vi "sub_create_buf_file_from_date.vi"(8 "error in (no error)":errorcluster) -> (0 "error out":errorcluster, 2 "new file path":path, 3 "File Refnum":refnum<file>)   [LabVIEW 2013, in "daqio minimal.lvlib"]
uses:
  daqio minimal.lvlib
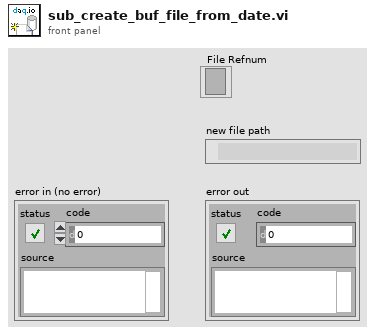
[diagram p1: front panel]
types:
  T1 = enum16{"open", "replace", "create", "open or create", "replace or create", "replace or create with confirmation"}
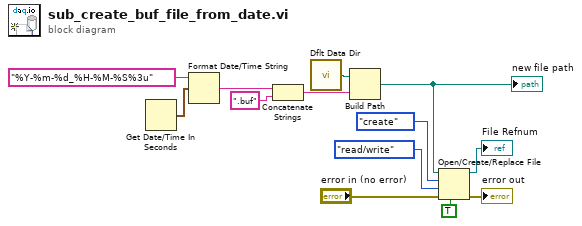
[diagram p0: block diagram]
diagram:
  n1 = Get Date/Time In Seconds() -> (seconds since 1Jan1904=w7:timestamp)
  n2 = Format Date/Time String(time format string (%c)="%Y-%m-%d_%H-%M-%S%3u", seconds (now)=w7) -> (date/time string=w9:string)  [unwired: 1 in]
  n3 = Concatenate Strings(w9, ".buf" ("string")) -> (w5:string)
  n4 = call <vilib>:"Dflt Data Dir.vi"() -> ("App:Default Data Directory"=w4:path)
  n5 = Build Path(base path=w4, name or relative path=w5) -> (appended path=w10:path)
  "new file path" <- w10
  n6 = Open/Create/Replace File(file path (use dialog)=w10, error in="error in (no error)", operation (0:open)=T1."create", access (0:read/write)=enum16{"read/write", "read-only", "write-only"}."read/write", disable buffering (F)=TRUE) -> (refnum out=→"File Refnum":refnum<file>, error out=→"error out":errorcluster)  [unwired: 1 in, 1 out]
